vi "Init_Action_1.vi"(8 "error in":errorcluster caption="错误输入（无错误）", 11 "AutoDetPort":bool) -> (0 "error out":errorcluster caption="错误输出")   [LabVIEW 2013]
uses:
  SystemCode/SysControl/Slot.ctl
  GlobalValue.vi
  <vilib>/Utility/error.llb/Error Cluster From Error Code.vi
  <vilib>/ErrorRing/Error Ring.xnode
  <resource>/objmgr/daqmx.rc
  InstrumentDrivers/USB-CAN/InitConfig.ctl
  InstrumentDrivers/USB-CAN/DevType.ctl
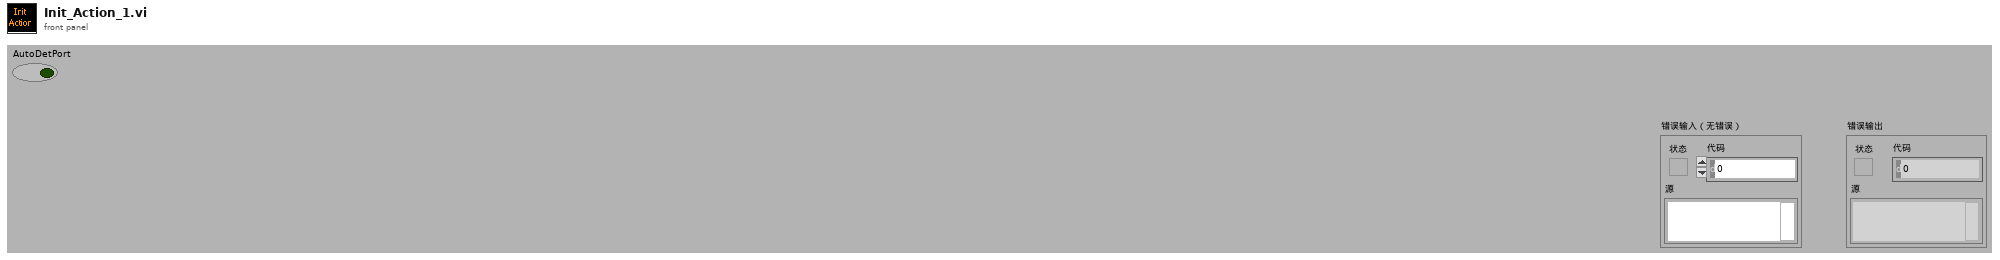
[diagram p1: front panel]
types:
  T1 = typedef "Slot.ctl" = enum16{"Slot1", "Slot2", "Slot3", "Slot4"}
  T2 = typedef "InitConfig.ctl" = cluster{"AccCode":u32, "AccMask":u32, "Reserved":u32, "Filter":u8, "kCanBaud":u8, "Timing0":u8, "Timing1":u8, "Mode":u8, "CanRx_IER":u8}
  T3 = typedef "DevType.ctl" = u16
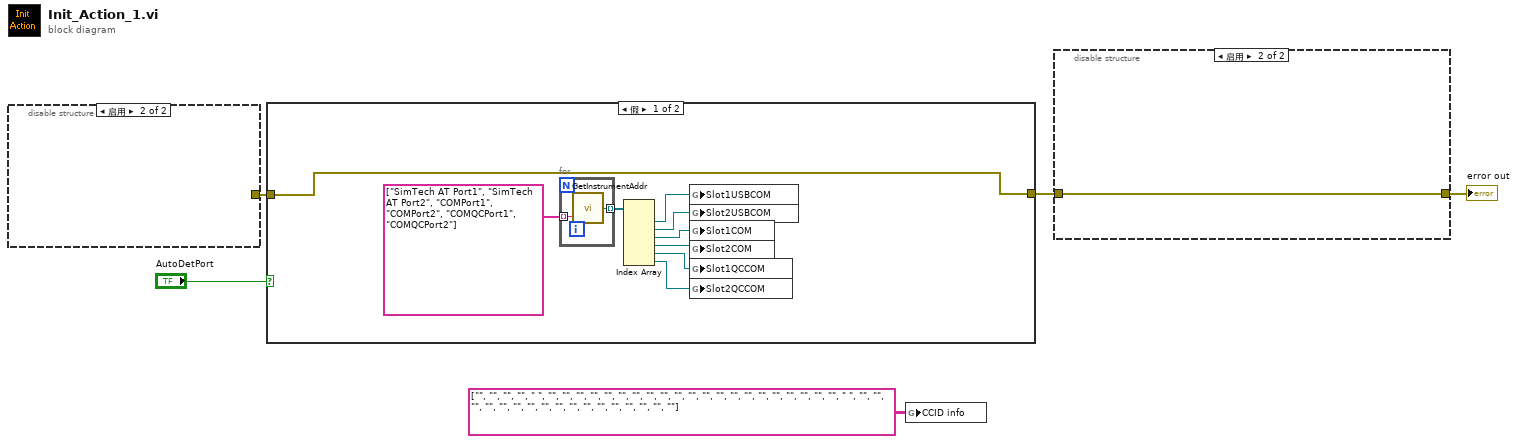
[diagram p0: block diagram]
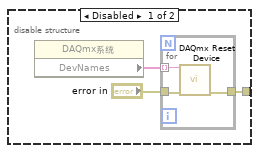
[diagram p2: hidden frame]
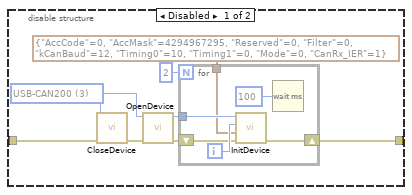
[diagram p3: hidden frame]
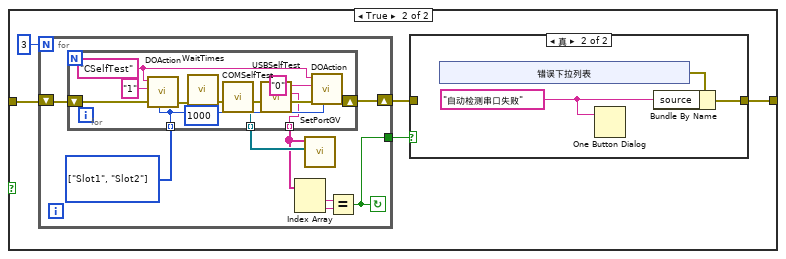
[diagram p4: hidden frame]
diagram:
  n1 = disable-structure shown="启用" {
    disable-tunnel: [w6 _] -> w5
    frame Disabled {
      n2 = property class="DAQmx系统"() -> ("DevNames"=w7:tag[])  [unwired: 2 in, 2 out]
      n3 = for {
        tunnel: [w10] -> w6
        tunnel: "error in" -> [w11]
        tunnel: w7 -> [w9] mode=indexing
        n4 = call <vilib>:"DAQmx Reset Device.vi"("device in"=w9, "error in"=w11) -> ("error out"=w10:errorcluster)  [unwired: 13 in]
      }
    }
    frame Enabled {
    }
  }
  n5 = case shown="假" "AutoDetPort" {
    tunnel: w5 -> [w14 w27]
    tunnel: [w14 w26] -> w3
    frame False {
      n6 = for {
        tunnel: string[] ["SimTech AT Port1", "SimTech AT Port2", "COMPort1", "COMPort2", "COMQCPort1", "COMQCPort2"] ("数组") -> [w22] mode=indexing
        tunnel: [w21] -> w19 mode=indexing
        n7 = call "GetInstrumentAddr.vi"("String"=w22) -> ("VISA session"=w21:refnum<visa-resource-name>)  [unwired: 1 out]
      }
      n8 = Index Array(array=w19) -> (element #1=w18:refnum<visa-resource-name>, element #2=w17:refnum<visa-resource-name>, element #3=w16:refnum<visa-resource-name>, element #4=w15:refnum<visa-resource-name>, element #5=w13:refnum<visa-resource-name>, element #6=w12:refnum<visa-resource-name>)  [unwired: 6 in]
      n9 = global write "GlobalValue.vi" "Slot1USBCOM"(w18) -> ()
      n10 = global write "GlobalValue.vi" "Slot2USBCOM"(w17) -> ()
      n11 = global write "GlobalValue.vi" "Slot1COM"(w16) -> ()
      n12 = global write "GlobalValue.vi" "Slot2COM"(w15) -> ()
      n13 = global write "GlobalValue.vi" "Slot1QCCOM"(w13) -> ()
      n14 = global write "GlobalValue.vi" "Slot2QCCOM"(w12) -> ()
    }
    frame True {
      n15 = for {
        N: 3 -> [_]
        shift-right: [w40] -> w23
        shift-left: w27 -> [w41]
        tunnel: [w36] -> w24
        stop <- w36 continue-if-true
        w43 = T1[] [enum."Slot1", enum."Slot2"] items=["Slot1", "Slot2", "Slot3", "Slot4"]
        n16 = for {
          tunnel: w43 -> [w54] mode=indexing
          shift-right: [w51] -> w40
          shift-left: w41 -> [w52]
          tunnel: [w50] -> w42 mode=indexing
          tunnel: [w47] -> w39 mode=indexing
          w53 = "CSelfTest" ("CH")
          n17 = call "DOAction.vi"("Slot"=w54, "error in"=w52, "State"="1", "CH"=w53) -> ("error out"=w46:errorcluster)  [unwired: 7 in]
          n18 = call "WaitTimes.vi"("WaitTimes"=u32 1000, "error in (no error)"=w46) -> ("error out"=w45:errorcluster)  [unwired: 9 in]
          n19 = call "COMSelfTest.vi"("error in (no error)"=w45) -> ("error out"=w49:errorcluster, "COMOUT"=w50:refnum<visa-resource-name>)  [unwired: 9 in]
          n20 = call "USBSelfTest.vi"("error in (no error)"=w49) -> ("error out"=w48:errorcluster, "USB"=w47:string)  [unwired: 8 in, 1 out]
          n21 = call "DOAction.vi"("Slot"=w54, "error in"=w48, "State"="0", "CH"=w53) -> ("error out"=w51:errorcluster)  [unwired: 7 in]
        }
        n22 = Index Array(array=w39) -> (element #1=w38:string, element #2=w37:string)  [unwired: 2 in]
        n23 = call "SetPortGV.vi"("COM"=w42, "USB"=w39) -> ()  [unwired: 10 in]
        n24 = Equal?(x=w38, y=w37) -> (x = y?=w36:bool)
      }
      n25 = case shown="真" w24 {
        tunnel: [w28 w29] -> w26
        tunnel: w23 -> [w28 _]
        frame False {
        }
        frame True {
          w30 = "自动检测串口失败" ("消息")
          n26 = xnode "错误下拉列表"() -> ("错误输出"=w31:errorcluster)
          n27 = One Button Dialog(message=w30) -> ()  [unwired: 1 in, 1 out]
          n28 = Bundle By Name(cluster=w31, "source"=w30) -> (w29:errorcluster)
        }
      }
    }
  }
  n29 = global write "GlobalValue.vi" "CCID info"(string[][] [["", "", "", "", " ", "", "", "", "", "", "", "", "", "", "", "", "", "", "", "", "", ""], ["", "", "", "", " ", "", "", "", "", "", "", "", "", "", "", "", "", "", "", "", "", ""]] ("CCID info")) -> ()
  n30 = disable-structure shown="启用" {
    disable-tunnel: [w60 w71] -> w4
    disable-tunnel: w3 -> [w59 w71]
    frame Disabled {
      w57 = T3 3 items=["PCI-CAN200"=7, "USB-CAN"=2, "USB-CAN200"=3] ("DeviceType")
      n31 = call "CloseDevice.vi"("错误输入（无错误）"=w59, "DeviceType"=w57) -> ("错误输出"=w58:errorcluster)  [unwired: 7 in, 2 out]
      n32 = call "OpenDevice.vi"("错误输入（无错误）"=w58, "DeviceType"=w57) -> ("错误输出"=w62:errorcluster, "DeviceTypeOut"=w64:u16)  [unwired: 7 in, 1 out]
      n33 = for {
        N: 2 -> [_]
        tunnel: w64 -> [w70]
        shift-right: [w66] -> w60
        shift-left: w62 -> [w67]
        tunnel: T2 {"AccCode"=0, "AccMask"=4294967295, "Reserved"=0, "Filter"=0, "kCanBaud"=12, "Timing0"=10, "Timing1"=0, "Mode"=0, "CanRx_IER"=1} ("InitConfig") -> [w65]
        i -> [w69]
        n34 = call "InitDevice.vi"("错误输入（无错误）"=w67, "InitConfig"=w65, "CanChannel"=w69, "DeviceType"=w70) -> ("错误输出"=w66:errorcluster)  [unwired: 5 in, 2 out]
        n35 = Wait (ms)(milliseconds to wait=u32 100 ("等待时间（毫秒）")) -> ()  [unwired: 1 out]
      }
    }
    frame Enabled {
    }
  }
  "error out" <- w4
